vi "FindVISA_UI.vi"() -> ()   [LabVIEW 2021]
panel:
  in  "VISA resource name":refnum<visa-resource-name>
  # "This simple VI can be used to see what connections are currently available by just opening the drop-down menu"
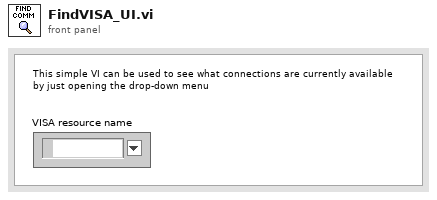
[diagram p1: front panel]
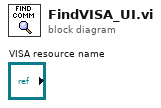
[diagram p0: block diagram]
diagram:
